vi "Run scan.vi"(4 "error in (no error)":errorcluster, 5 "file path":path, 6 "Position List":sgl[][](array[numeric]), 7 "Controller Reference In":refnum<k7>) -> (0 "error out":errorcluster, 1 "file path out":path, 3 "Controller Reference Out":refnum<k7>)   [LabVIEW 2015]
panel:
  in  "VISA resource name":refnum<visa-resource-name>="COM4"
  in  "Stop":bool
  in  "Speed":sgl=100.0
  # "X Axis"
  # "Y Axis"
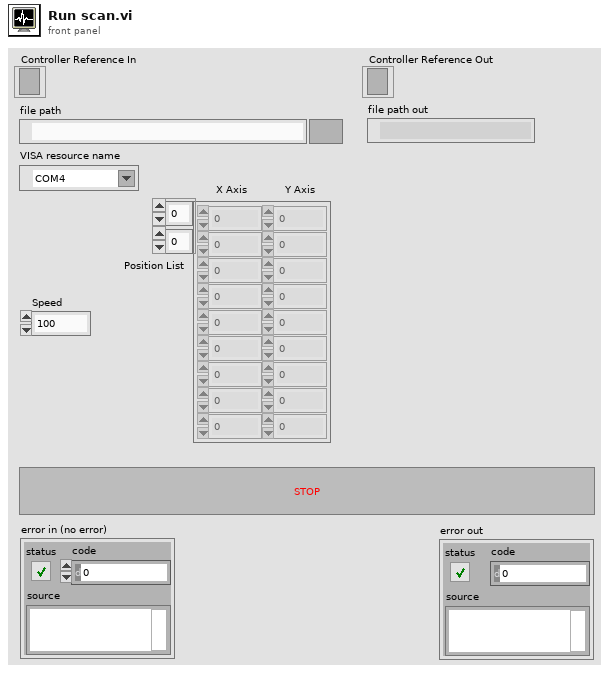
[diagram p1: front panel]
types:
  T1 = enum16{"open", "open or create", "create or replace", "create", "open (read-only)"}
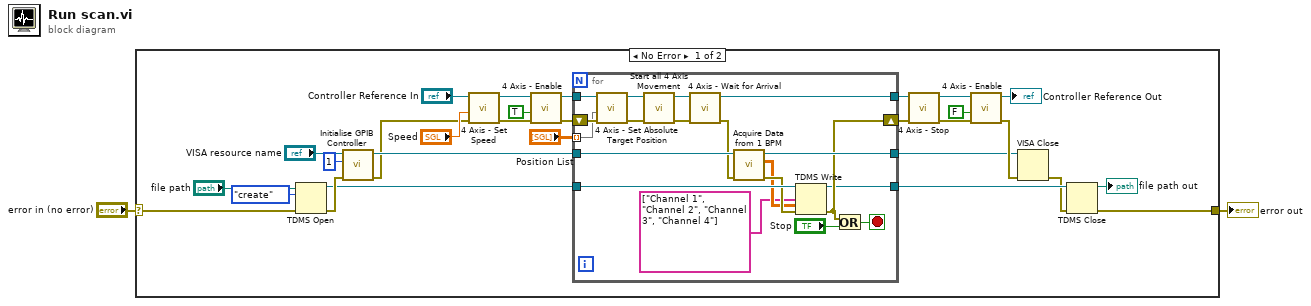
[diagram p0: block diagram]
diagram:
  n1 = case shown="No Error" "error in (no error)" {
    selector: "error in (no error)" -> [w8 w51]
    tunnel: [w9 w51] -> w2
    frame No Error {
      n2 = TDMS Open(8:w8, 10:T1."create" ("operation (0:open)"), 11:"file path") -> (0:w14:errorcluster, 3:w13:refnum<k34>)  [unwired: 4 in]
      n3 = call "Initialise GPIB Controller.vi"("error in (no error)"=w14, "Address"=u32 1, "VISA Refnum In"="VISA resource name") -> ("error out"=w6:errorcluster, "VISA Refnum out"=w30:refnum<visa-resource-name>)  [unwired: 3 in]
      n4 = call "4 Axis - Set Speed.vi"("error in (no error)"=w6, "Speed"="Speed", "Controller Reference In"="Controller Reference In") -> ("error out"=w25:errorcluster, "Controller Reference Out"=w26:refnum<k7>)  [unwired: 3 in]
      n5 = call "4 Axis - Enable.vi"("error in (no error)"=w25, "Enable/Disable"=TRUE, "Controller Reference In"=w26) -> ("error out"=w23:errorcluster, "Controller Reference Out"=w22:refnum<k7>)  [unwired: 3 in]
      n6 = for {
        tunnel: "Position List" -> [w47] mode=indexing
        tunnel: w30 -> [w50]
        tunnel: w22 -> [w48]
        tunnel: [w41] -> w21
        tunnel: [w40] -> w15
        tunnel: w13 -> [w37]
        tunnel: [w34] -> w11
        shift-right: [w35] -> w20
        shift-left: w23 -> [w49]
        stop <- w38 stop-if-true
        n7 = call "4 Axis - Set Absolute Target Position.vi"("error in (no error)"=w49, "Positions"=w47, "Controller Reference In"=w48) -> ("error out"=w45:errorcluster, "Controller Reference Out"=w46:refnum<k7>)  [unwired: 3 in]
        n8 = call "Start all 4 Axis Movement.vi"("error in (no error)"=w45, "Mint Controller reference In"=w46) -> ("error out"=w43:errorcluster, "Mint Controller reference out"=w44:refnum<k7>)  [unwired: 4 in]
        n9 = call "4 Axis - Wait for Arrival.vi"("error in (no error)"=w43, "Controller Reference In"=w44) -> ("error out"=w42:errorcluster, "Controller Reference out"=w41:refnum<k7>)  [unwired: 4 in]
        n10 = call "Acquire Data from 1 BPM.vi"("error in (no error)"=w42, "VISA resource in"=w50) -> ("error out"=w36:errorcluster, "BPM Values"=w33:dbl[][], "VISA resource out"=w40:refnum<visa-resource-name>)  [unwired: 3 in]
        n11 = TDMS Write(0:w37, 7:string[] ["Channel 1", "Channel 2", "Channel 3", "Channel 4"] ("channel name(s) in (Untitled)"), 9:w33, 11:w36) -> (4:w34:refnum<k34>, 15:w35:errorcluster)  [unwired: 2 in, 2 out]
        n12 = Or(x=w35, y="Stop") -> (x .or. y?=w38:bool)
      }
      n13 = call "4 Axis - Stop.vi"("error in (no error)"=w20, "Controller Reference"=w21) -> ("error out"=w18:errorcluster, "Controller Reference out"=w19:refnum<k7>)  [unwired: 4 in]
      n14 = call "4 Axis - Enable.vi"("error in (no error)"=w18, "Enable/Disable"=FALSE, "Controller Reference In"=w19) -> ("error out"=w16:errorcluster, "Controller Reference Out"=→"Controller Reference Out":refnum<k7>)  [unwired: 3 in]
      n15 = VISA Close(VISA resource name=w15, error in (no error)=w16) -> (error out=w10:errorcluster)
      n16 = TDMS Close(8:w10, 11:w11) -> (0:w9:errorcluster, 3:→"file path out":path)
    }
    frame Error {
    }
  }
  "error out" <- w2
